vi "_Read Modules to Launch.vi"(8 "error in (no error)":errorcluster, 11 "launcher in":refnum<class "launcher.lvclass">) -> (0 "error out":errorcluster, 2 "Modules to Launch":T1[](array[typedef]), 3 "launcher out":refnum<class "launcher.lvclass">)   [LabVIEW 2021, in "launcher.lvclass"]
uses:
  launcher.lvclass
  <userlib>/S2 Labs/Module Framework/Modules/Base/Launch Module Typdef.ctl
  <userlib>/S2 Labs/Module Framework/Modules/Base/Launch Module Parms.ctl
  launcher.lvclass/launcher.ctl
  <userlib>/S2 Labs/Module Framework/Modules/Base/Module.lvclass
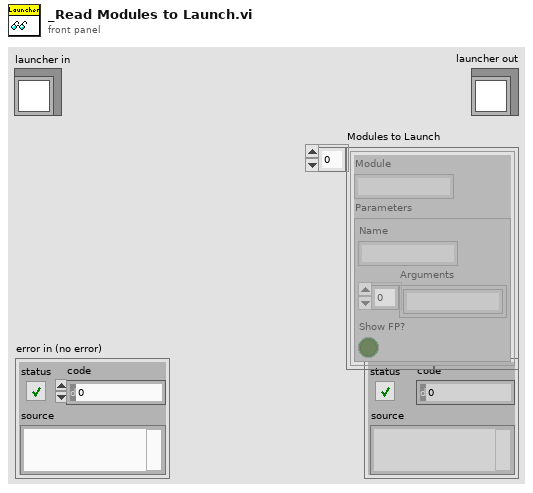
[diagram p1: front panel]
types:
  T1 = typedef "Module.lvclass/Launch Module Typdef.ctl" = cluster{"Module":string, "Parameters":T2}
  T2 = typedef "Module.lvclass/Launch Module Parms.ctl" = cluster{"Name":string, "Arguments":string[], "Show FP?":bool}
  T3 = typedef "launcher.lvclass/dvr_type.ctl" = cluster{"_PARMS":T4}
  T4 = typedef "launcher.lvclass/_PARMS.ctl" = cluster{"ch_alias":string[], "ch_units":string[], "Modules to Launch":T1[]}
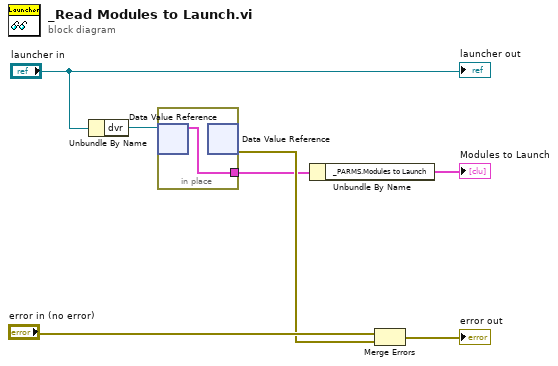
[diagram p0: block diagram]
diagram:
  n1 = Unbundle By Name ("DVR Unbundle")("launcher in") -> ("dvr"=w3:refnum<data-value>)
  n2 = in-place "In Place Element Structure" {
    in-place-border: [w8] -> w2
    n3 = in-place-dvr #1(w3) -> (w8:T3)  [unwired: 1 out]
    n4 = in-place-dvr #1() -> (w4:errorcluster)  [unwired: 1 in, 1 out]
  }
  n5 = Unbundle By Name ("Item Unbundle")(w2) -> ("_PARMS.Modules to Launch"=→"Modules to Launch":T1[])
  n6 = Merge Errors("error in (no error)", w4) -> (→"error out":errorcluster)
  "launcher out" <- "launcher in"
